vi "Name Value AutoComplete Items.vi"(0 "Input String":string, 2 "Match Limit":i32=-1, 5 "Sorted Tags":string[](array[string]), 7 "First Letters":string[](array[string]), 9 "Letter Indicies":i32[](array[numeric])) -> (8 "AutoComplete":string[](array[string]))   [LabVIEW 2020]
uses:
  24645ac3-8699-421e-a56c-b73a1a18a263.vi
  24645ac3-8699-421e-a56c-b73a1a18a263.vi/d4db2432-cc9c-482c-8957-dac855435ef6.vi
  24645ac3-8699-421e-a56c-b73a1a18a263.vi/86fbf154-bd7b-49a2-8ab2-a837b2a95f24.vi
  24645ac3-8699-421e-a56c-b73a1a18a263.vi/3b95b01e-1ec2-4565-bcd9-7606a5281010.vi
  24645ac3-8699-421e-a56c-b73a1a18a263.vi/96a08935-737a-44b2-979c-a81d56408f7e.vi
  24645ac3-8699-421e-a56c-b73a1a18a263.vi/d4db2432-cc9c-482c-8957-dac855435ef6.vi/6eaecd13-6e48-4772-a921-b51ebdf84d88.vi
  24645ac3-8699-421e-a56c-b73a1a18a263.vi/d4db2432-cc9c-482c-8957-dac855435ef6.vi/d2d5f2b7-06f4-47f6-971c-049c3fdbb653.vi
  24645ac3-8699-421e-a56c-b73a1a18a263.vi/3b95b01e-1ec2-4565-bcd9-7606a5281010.vi/6eaecd13-6e48-4772-a921-b51ebdf84d88.vi
  24645ac3-8699-421e-a56c-b73a1a18a263.vi/3b95b01e-1ec2-4565-bcd9-7606a5281010.vi/d2d5f2b7-06f4-47f6-971c-049c3fdbb653.vi
  24645ac3-8699-421e-a56c-b73a1a18a263.vi/96a08935-737a-44b2-979c-a81d56408f7e.vi/6eaecd13-6e48-4772-a921-b51ebdf84d88.vi
  24645ac3-8699-421e-a56c-b73a1a18a263.vi/96a08935-737a-44b2-979c-a81d56408f7e.vi/d2d5f2b7-06f4-47f6-971c-049c3fdbb653.vi
  <vilib>/Comparison/Less/Less Functor/Less Functor.lvclass
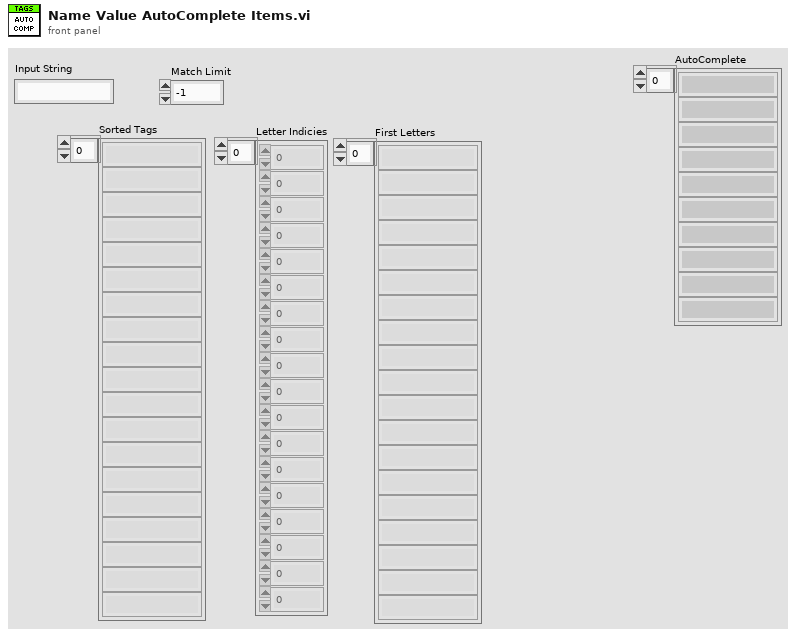
[diagram p1: front panel]
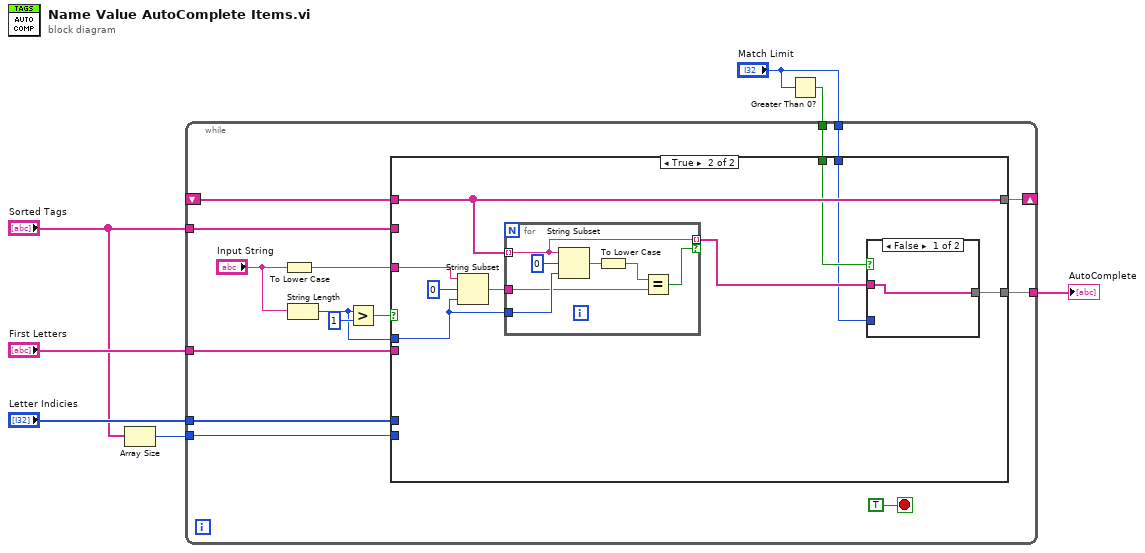
[diagram p0: block diagram]
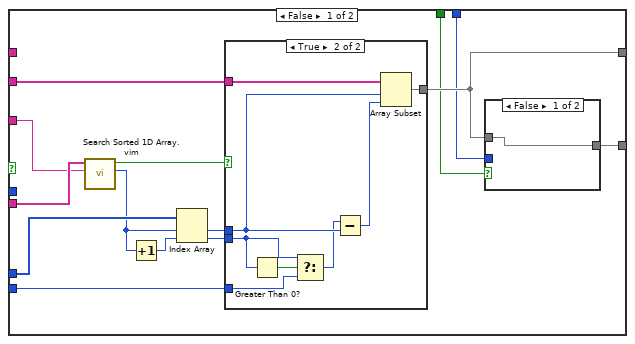
[diagram p2: hidden frame]
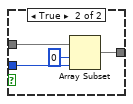
[diagram p3: hidden frame]
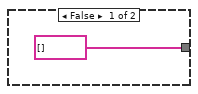
[diagram p4: hidden frame]
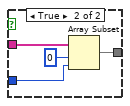
[diagram p5: hidden frame]
diagram:
  n1 = Array Size(array="Sorted Tags") -> (size(s)=w4:i32)
  n2 = Greater Than 0?(x="Match Limit") -> (x > 0?=w1:bool)
  n3 = while {
    tunnel: "First Letters" -> [w21]
    tunnel: "Letter Indicies" -> [w20]
    tunnel: "Sorted Tags" -> [w19]
    tunnel: w4 -> [w18]
    shift-right: [w17] -> _
    shift-left: _ -> [w16]
    tunnel: [w11] -> w3
    tunnel: "Match Limit" -> [w9]
    tunnel: w1 -> [w8]
    stop <- TRUE stop-if-true
    n4 = To Lower Case(string="Input String") -> (all lower case string=w13:string)
    n5 = String Length(string="Input String") -> (length=w10:i32)
    n6 = Greater?(x=w10, y=1) -> (0:w14:bool)
    n7 = case shown="True" w14 {
      tunnel: w21 -> [w36 _]
      tunnel: w20 -> [w35 _]
      tunnel: w19 -> [w30 _]
      tunnel: w18 -> [w28 _]
      tunnel: w13 -> [w27 w58]
      tunnel: [w26 w59] -> w17
      tunnel: w16 -> [_ w59]
      tunnel: w10 -> [_ w55]
      tunnel: [w25 w53] -> w11
      tunnel: w9 -> [w24 w51]
      tunnel: w8 -> [w23 w52]
      frame False {
        n8 = call "Search Sorted 1D Array.vim"("element"=w27, "sorted 1D array"=w36) -> ("nearest index"=w33:i32, "found?"=w31:bool)  [unwired: 8 in]
        n9 = Increment(x=w33) -> (x+1=w32:i32)
        n10 = Index Array(array=w35, index #1=w33, index #2=w32) -> (element #1=w34:i32, element #2=w29:i32)
        n11 = case shown="True" w31 {
          tunnel: w34 -> [_ w48]
          tunnel: w30 -> [_ w50]
          tunnel: w29 -> [_ w45]
          tunnel: w28 -> [_ w46]
          tunnel: [string[] [] w43] -> w26
          frame False {
          }
          frame True {
            n12 = Greater Than 0?(x=w45) -> (x > 0?=w47:bool)
            n13 = Select(t=w45, s=w47, f=w46) -> (s? t:f=w44:i32)
            n14 = Subtract(x=w44, y=w48) -> (x-y=w49:i32)
            n15 = Array Subset(array=w50, index=w48, length=w49) -> (w43:string[])
          }
        }
        n16 = case shown="False" w23 {
          tunnel: w26 -> [w37 w41]
          tunnel: [w37 w39] -> w25
          tunnel: w24 -> [_ w38]
          frame False {
          }
          frame True {
            n17 = Array Subset(array=w41, index=0, length=w38) -> (w39:string[])
          }
        }
      }
      frame True {
        n18 = String Subset(string=w58, offset (0)=0, length (rest)=w55) -> (substring=w56:string)
        n19 = for {
          tunnel: w59 -> [w67] mode=indexing
          tunnel: w56 -> [w69]
          tunnel: w55 -> [w71]
          tunnel: [w67] -> w54 mode=indexing if=w66
          n20 = String Subset(string=w67, offset (0)=0, length (rest)=w71) -> (substring=w68:string)
          n21 = To Lower Case(string=w68) -> (all lower case string=w65:string)
          n22 = Equal?(x=w65, y=w69) -> (x = y?=w66:bool)
        }
        n23 = case shown="False" w52 {
          tunnel: w54 -> [w60 w64]
          tunnel: [w60 w62] -> w53
          tunnel: w51 -> [_ w61]
          frame False {
          }
          frame True {
            n24 = Array Subset(array=w64, index=0, length=w61) -> (w62:string[])
          }
        }
      }
    }
  }
  "AutoComplete" <- w3
